vi "day 17 task 1.vi"() -> ()   [LabVIEW 2019]
uses:
  day 17/day 17 data--cluster.ctl
panel:
  out "height":i32
  out "already fallen rocks max y":i32
  out "jet pattern index":i32
  out "action":enum16{"spawn rock", "jet", "try fall"}(ring)
  out "direction of jet":string
  out "visualisation":bool[][](array[boolean])
  out "transposed array":bool[][](array[boolean])
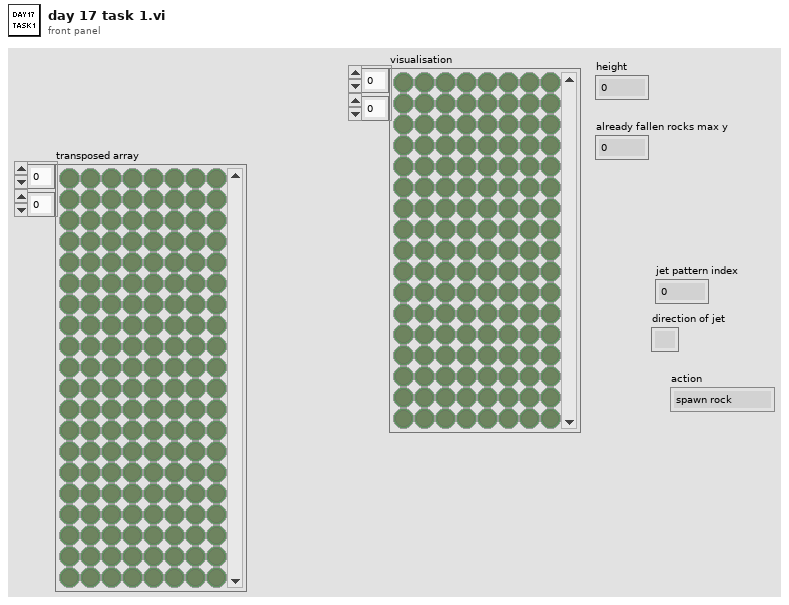
[diagram p1: front panel]
types:
  T1 = typedef "day 17 data--cluster.ctl" = cluster{"rock shape coords":cluster{cluster{"x":i32, "y":i32}[]}[], "index of next rock shape":i32, "currently falling rock's co-ords":cluster{"x":i32, "y":i32}[], "already fallen rocks' co-ords":cluster{"x":i32, "y":i32}[], "jet pattern":string, "index of next jet pattern index":i32, "next action":enum16{"spawn rock", "jet", "try fall"}, "already fallen rocks max y":i32, "no. rocks fallen":i64}
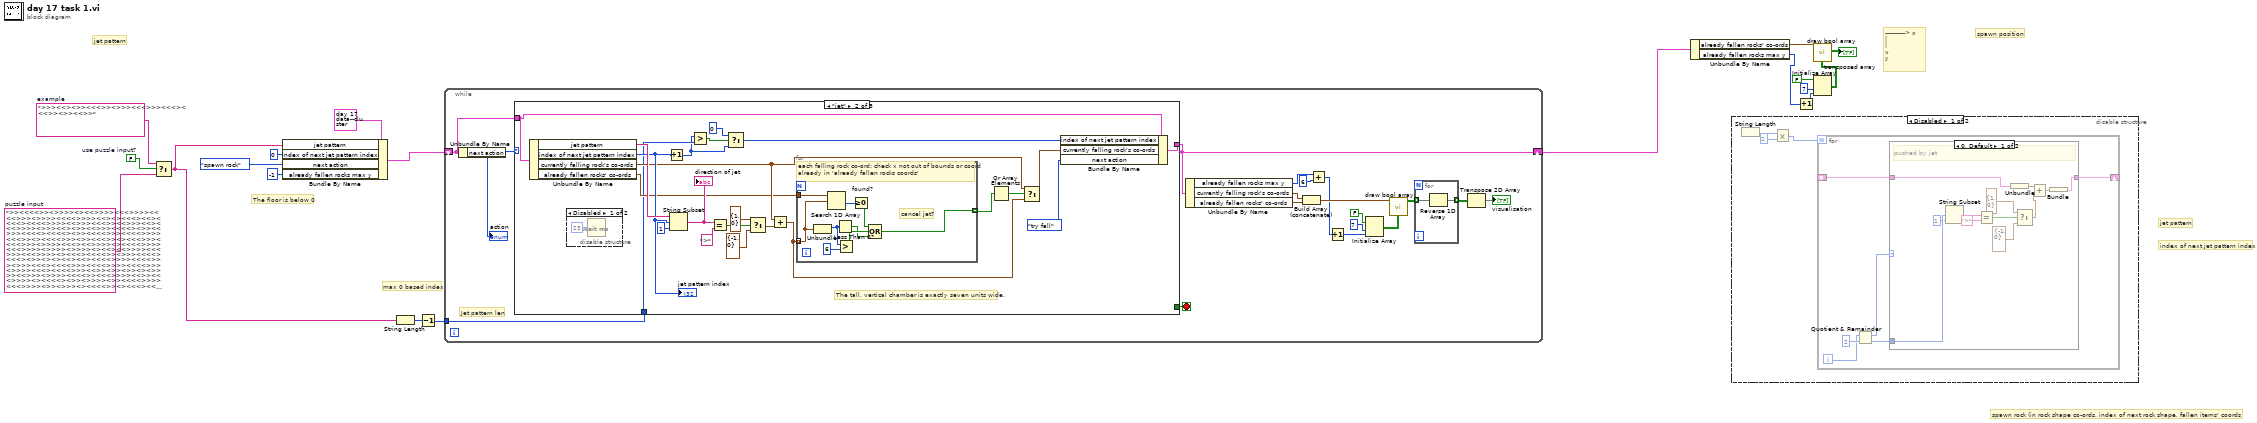
[diagram p0: block diagram]
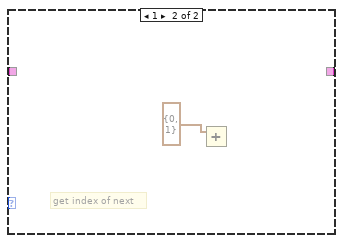
[diagram p2: hidden frame]
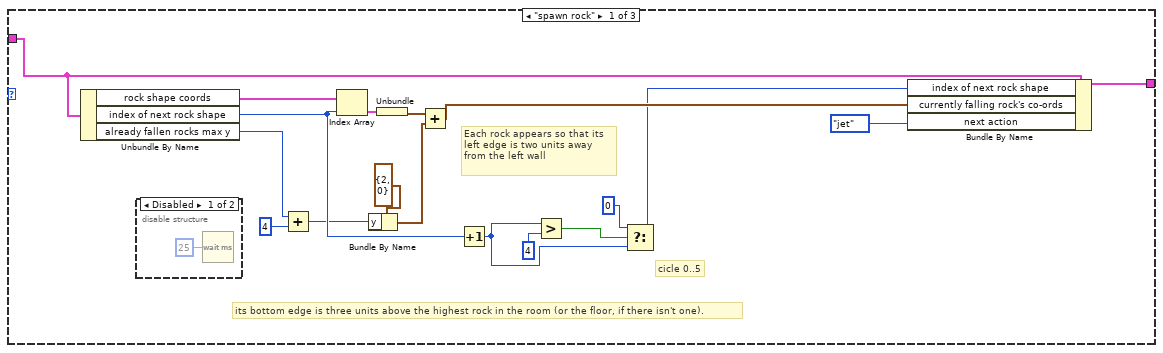
[diagram p4: hidden frame]
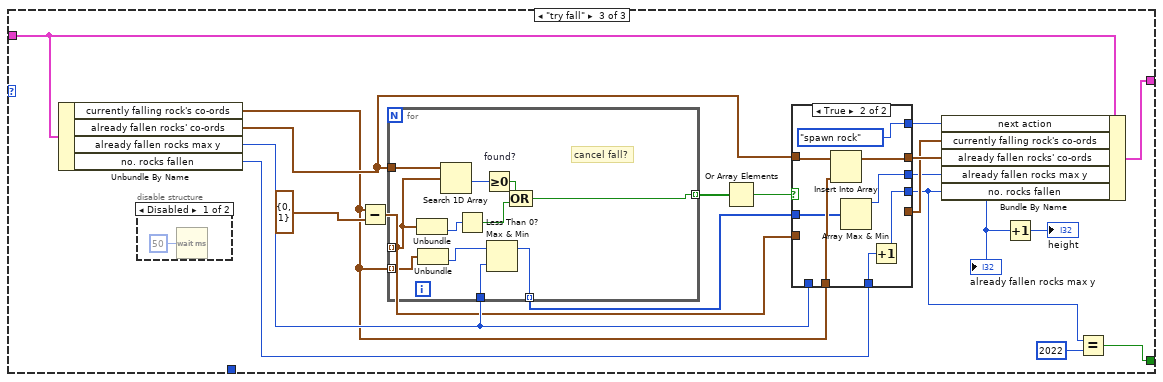
[diagram p7: hidden frame]
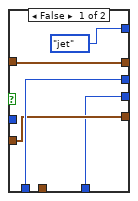
[diagram p8: hidden frame]
diagram:
  w17 = FALSE  # use puzzle input?
  w18 = ">><<<<>><>>>><><<>>>><<<>>>><<<<>>><>>>><<<<>>>><<><><<<><<><<<<><<<<>>>><<>>><<<>><<>>><<><<<>>>><>>><<><>><<>>><<<<><>><<>>><<<<><<<<><>><<<<>>><<<<>>>><<<>><><<<<>>><>><<<>><><<<>>><<<<>>><>>>><<<><<>>>><><<<<>>>><<<>>>><>>>><>>>><><<><<>>>><<<>>><<<>>>><><<<><<<<>><>>><<<<><<<><>><><><<><<><<<<>>>><<<<>>><>>><<<><<<<>>><<<<>>>><<<<>>><>>>><<<><<<<>>><<>><>><>><><>>>><<>>><>>>><<<<>><<<>>>><<>><<<>>>><><<<<><>><>>>><>><<<<>>>><<<>>>><>><>>><><<<<>><><<<><<<<>>><<><<<>>><<<<><<>>><<>><<<<><<>>>><<><>>><<><<<>>><<<<><<<<>><>>><<<>>><<<<>>>><<><<>><<<>><<>>>><<<>>>><<>><<>><<><<<<>><<<<>>><<><<<<>>><>><<>><<<<><<<><<<>>>><<<<>><>>>><<<<>><<>>><<>>>><<<<><<<><<>>><>>><<<>>>><>><<><><<<<>>>><<<<>>>><<<<><<<>>><<>><>>>><>>>><<<<>><<<<><<><>><<<<>><<<>>>><<>>>><<<<><<<>>><<<<>>><<>>><<<>>><<><<><<<>>><><<>>><<<>>>><>>>><<<><<<<><<>><><<>>>><><<<<>>><<><<<<><<<<><<<<>>>><<>><<<><<<>><<>>><<>><<<<><<><<<>>><<>><<<><>><<><<<<><<<<>><<>><<><>>><>>><<<>><<<>>>><>>><>><<><<>><><<<<><<<<>>><<<<>>><<<<><<<>>><<<>>>><<<>><<>><><<><<<<><>>>><>>>><<<<><>>><<<>><<<>>>><<<<>><<<<>><<<<>>>><>><<>>>><<<>>><<><<<>>>><<<><<><<<>>>><<<>>>><<>><<<<>>>><><<<>>><>>>><<<>>>><<>><<<<>>>><><<<>><<<>>><<>>><>>>><<>>><><<<<><>>>><><<<<>>>><<<<>><<<>>>><<<>><<<>><<<>>>><><<<<>>><<>>>><<>><><<<>>><<<>><<<>>>><>>>><<>>><<<<>>><<<>><><<<>>><<<<>>>><<>><<>>>><<<<>>><<<><>>><<<>>>><<<<>><<<<><<<<><<<<>>><<<>>><<<>>>><><>>>><>>><<>>><><>>><<>>><>><><<<>>>><<<>><<<<>>><<>>>><<>>><<<>><<<<>><>>><<<>>>><<<>>><<<>>><><><<<>>><<<>><<<>><<<<>><>>><<><>>><<>>><<>>><<<><>>><<<<>>><<<>>><<<>>><>>><<>><<>>>><><<<<>><>>>><<<<><<><<<<>>><>><>>>><<>>>><<>>>><<<>><>>><><<<<>>><><<>><<<>><<<<><<<><<<<><<<>><<>>>><<<<>>><>>><<<<><<<>><<<>>><<>>>><<<<>>>><<>>><><><<<<>>>><>>>><<<<>>><><<<><<<>>><>>><<<<><<<<><>>>><>>>><<><<<>>>><<>>><>>><<<<>>><<<<><<>>>><<<>>><<<<>>><>><<<><>>>><<>>><<<>><<<<>>>><<<>>><<<<><<<<><<>><>>><>><<<<><>>><>>>><<>><>>><<><<<><<>><<<>><>>><<<<>>>><>>>><<<<>>><<<><<<<>>>><<<<>>><<<<>>>><>>><<<>><<>>>><<<<>>>><<<<><<>>>><<<>><>>><<>><><<<<>><<<<>>><<<><<>>><>><<<><>><<>>><>>>><<>>><>>><>><<<><<>>>><<<<><<>><<<<><<<><<<<>>><<<<>>><<<>><<<<>>><<<<>>>><<><<>>><<<<><<>><<<<><<><<<<>>>><<<><<<<>><<<<><>>>><<><<<<>><>>>><><<<>>>><<<>><<<<>>>><<><<<<>><<>><<<<><<<><<>>><<>><>><<><<><>><<<<>>><<>>><>>><<<><<<<><<>>>><<>>><<>><>>>><><<<<><<>><>>><><<>>><<>>>><<<<>>><<<<>>>><<<>><<<<><<<>>><<<>><<<<><<<><><<>>>><<<>>>><<<>>>><<<>>><<>>>><<>>>><<<<>>><<>>><<<>><<>><<>>>><<<>>>><<<<><<>><>>><<<<>>>><<<><<>><>>>><>>>><>>>><<>><<<><<><>><<<>><<<<>><><<>><<>><<>>><><<<>><>><<><<<<><>>><>><<<>>>><<<>>><>>>><<>><><<>><<>>>><<<<><>>>><<>><<>>><<<>>>><<<<>><<>>><<<<>>>><>>><<<>><<<<>>>><<<<>>><<<>><<>>>><<<><<<<>><<<<>><<><<<>>><<>><<<><<<>>>><<<<>>>><<<<>><<<<>><><<>><<<<>>>><<<<>><<>>>><<>><>>>><<<><>><<><>><<>><><<><>>><<<>>>><>>><<>><>><>>>><<<<><<>><<<<><>>>><<>>><<>>><<><>>>><>><<<><<<><>>>><><<><<<<><<><<<<>>>><><<<<>>>><<<>><<>><<<<>>>><<<<>>>><<<>>>><>>><<<>>>><<<>><<<<>>>><<<>><<>>><<<<>>><<><<<<>>>><>><<<>><<>>>><<<<>>>><<>>><<<<>><><<<<>>><<<>>>><<>>>><><>>>><<>>><>>><<<>>><<<>><<<>><<<<><><<><<<<>><>>><>>><><>>><<<>>><<>><<><<<>>>><<<>>><>><><<>>>><<<><>><<<<>><<<><>>><<><<<<>>>><<>>>><<<<>><<<<>><<<<>>>><<<<>>><<<<><<<>><<>><<<<>><<><<<<>><<<<>>><<<<><<<<>>>><<><<<><<<<>>>><<>>><<<<>>>><<<<><<>>><>>><<<><<<<>><<<>>><>>>><><>>>><><>>><<<>>>><<<><>>>><<<>><<<><<>><<><><<<<><<>>><<>><<><<<>>>><<<>>><>>><>><<<<>>><<><<<<>><>>><<<>>>><<>><>>><<<>>><<<>><<<<>>>><>>><>>>><>>><<<>>><<<>>>><<<>><<<>><<<><><>>>><<<<>>>><<<<><>>><><<<<>>><<<<>>><<><><><<>><<><<<<>>><>>>><<>>><<>>>><<<>>><<<>><<<<><>>><>><<<<><<>><<<<><<<<>>>><<<>>><>>>><<<<>>>><<<<><<<<>>>><<<<>>>><<<>><<<<>>>><<>><<<>>>><<<>>>><<<<>><<<><>>>><<><>>>><<<<><>>><><<<><>>>><<>><<<<>><>><<<<>>>><<<<>><<>>><><<<><<<<>>>><>>>><<>><<<><<>>><<>><>><<>><<><<<<>><>><<<<>>>><<<<>><<<<>>><<><<>><>>><<<<>>>><<>>>><<><<>>>><<>><<>>>><<<>><<<<>>>><>>>><<<<><<<><><<<><<<<>><<<><<>><<<<>><<<<>>><<<><<<>><<>><<<>>><<><<>><<>>><<<>>>><>>><<<>>>><<>>><<<<>>>><><>>><<<<>>>><>>>><<<>>><<>>>><<<>><>><>><<<>>><<<>>>><<<>>><<<>>>><<>>>><<<><>><<>>><<<<>>>><><<<<><<>><>><>>><>>>><<>>><<<<>>><<<<><<<>>>><<<<>>>><<<<>>><>><>><<<<>>><<<<>>>><<>>>><<<<><>><<>>>><>>><<>><<<>>><<<>><<<><<<<>>>><<<<>><<>><<>>>><<<<>>>><>><<>>><<<<><<<><><<<>>><<>>><<<>>><<<>><<>>><>><<<>>>><<>>>><<<<>>>><<>><>>>><<<<><>>><<<<>>>><<>>>><<<<>>><<<<>>><<<<>><<>>><<>>>><<>>><<<><<<>>><<>>>><<<<><<>><<<<>>>><>>>><>><><<><<><<<<>><<<><<>>><>>><>>><<<<><<<<><<<<>>>><<>><>>><>>><<<><>>>><>>><>>><<<>><<<><<<>><<<<>>>><<<>>>><<<>><>><<>><<<>>>><<<<>>>><<<>>><><>><<><<<>><<<<>>><<>><<>><<<<>>><<<>>>><<>>>><<<<>>><<<>>><<<><>>>><<<<>><>><<<<>>>><<>>><<<>><><<<><<<<><>>>><>><><>><<<>>>><<<>>><<>>>><><<<<><<<>><<<<>>><<<><<><<<>><>>><><<<>>>><<<<>>>><<<>><>><<<>><<<>><<><<<<>>>><<>>><<<>>><>>>><<<>><<<<>>><<><>><<<<><<<<>><<<>><><>><<<><<<><><<<<>>>><<<><<<<><<<>>>><<>><<><><>>>><><>>><<>>><<<>><<<><<<<>>>><<<><<>><<<<>>><>><<><<>>>><<<>>><<<><<<>>><><<<<>>>><<><>><>>><<>>><<>>>><<>>><<>>>><>><><<<<>><>>><<<>>><<<>><<>>><<<<>><>>><<>>>><<<>>><>>><<<>><<<><<<>>><<><<<>>>><<>><<<<>>><<<>>><<<>>>><>><<<>>><<<<>>>><<><>>>><>>>><<<<>><<<>>>><>>>><<<>><<<<>><<><<>>>><<<<>>><<<<>>><<>><<<<>><<>>><<>>>><>><<>>><<>>>><>>>><>>><<<><<>><<<<>>>><<<>><<<<>>>><<<>><<<><<<>>><<<>><>>><<<<>>>><>>>><<<>><<<<>>><>>>><>><<><><><<<<>>>><<<<><>>><<>><<<>><<<>><<><<>><>><<<><<<>><<<>>><<<>><<>>><<<>>><<<<><>>><>>>><><<>>>><>>>><<<<>>><>>><<<<>>><>>>><>>>><<<<>>>><<>>>><<<>>><<>><<>>><<>>>><<>><>>>><<<>><<<><<><<<>><<<<>>><<>>>><<<<><>><<<>>>><<<>>>><<>><<>>>><<><>><>>><<<<>><<<>>>><<<>>>><<<<>>>><>>>><>>><<<<>>>><<<<><<>>>><<<<>>><<<<>><<>><>>><<<>><<<><<<<>>><><>><>>>><><<><<<<>>>><><<<>><<>>><<<<>>><<<<><>>><<>><>><<<><><>><<>>><<><><<><>><<>>>><<<<><<>><<<><<<><<>>><<<<><>><>>><<<><<<>><<><<<>><<<<>>>><<<>>><<>>>><><>><>>>><>>><>>>><>>><<<<>>>><<<>>><<<<>>>><>><<<<><<>><>><<>>><<<<>>>><<<>>><<<>><<<>><<>><<<<><>>>><>>>><<>>><<<><>><>><<<<>>><>>>><>><<>>>><<<<>><>>><<>>><<<<>>>><<><<<<>>>><<><<>><><>>>><>>><>>>><>>><<><>>><<>>><<<>>><<<<>>>><>>><<>><>><>>>><<>><<<>>><<<>>>><>><<>>><<>>><<><<>>>><<<<>>>><>><<<<>>>><<<<>>>><<>><<>>>><<<<>>>><<<<>><>>><>>>><<<>><>>>><<<><<>>>><<>>><<>>>><<><<<><<<<><<<>>><<>>><<<>>>><<><<<><><<>><<<<><<<<>>><<><<<<>><<<<>>>><<<>>>><<<>><<<<>>><>>><<<<>>><<<>>><<<<>><<<<>>><<>>><<<>><<<<>>><>>><<<>><<<<><<<<>>><<><<<<>>>><<<>>>><<>>><<><<<>>>><>>>><<>>>><>><<>><<>>>><<<<>>><<<>>>><<><<<><>><<<<>>><><>><<>>><<<>><<<>>><<<<><<<>>><<<<>>><<<<>><<><<<<>>>><<<><>><<>><>>>><>><<>><><<<>><<<>><<<<>>>><<<>>><<><<>>>><<>>>><<>>><<>><<<<>>>><<<<>><<>>>><<<>>>><<<<>>><<><<<<>>>><<<><>>><<<>><><>>>><><<<>>>><<<<>><<>><<<>><<><<><<<<>><><<<<>>><<><<>><<<>>>><<<>>><<>>><<<<>><<><<<<>>><<<<><><<<>>><<<><<<<>>><<<<>>><<<<>>><<<<>>><<>>><<<<>>><>><<<>><<<<>>>><><>>>><<><<><<<<>><><<<>>><><<<><<<>>>><<>><<<<>>><<<<><<<>>>><<>>>><<<<>><<<>>>><>>><<<>>>><<<>>>><<<>>><>>>><<<<>><>><<>><><<<<><<<>>>><<<>>><>>>><>>>><<<><<<>>><<>>>><>>><><<<<>><<>>><<<>><<>>><<<<><<<<>>>><<><<<><>>>><<<>>><<>>>><<<<>>>><<<<>>>><>><<<<>>><>>>><<>>>><<<><<>><<<>>><<<><<>>><<<<>>><<<<><<>>>><<>><<<>>><<<<>><<><<<<>>>><<><<>>><<<>>>><<<><<>><<<>>>><<><<>>>><>><<<<>>>><<>><>><<>>><<<><<<<><<<<>>><>><><>>><<<>>><<>><><<>><<<>>><<<>><<<<>>><<<<><<<><>><>>><<<<>>>><<<<>><<<<>><>>>><>>>><>>>><<<<>><>>>><<>><<<>>><<>><><>>>><<><<<<>><<>>><<>>><<>>><<<<>>>><<<<>><<<>>><<><<<<>><<<<>><<><>>>><<<>>>><<<><<>><<<<>>><<<<><>>>><<<<>>>><<>>>><<>><>>><>>><<><<<<>><<<<>><><<>><>><>>><<><<<>>>><<<>>><<<<>>>><<><<><>>><<<<><><<>>>><<<<>><<<<>><<>><<>>>><<>>>><<>>><<<>>>><<>>>><<<<>><>><>><<>>>><<<>>>><<<<>><<<>>><<>>><<<<>>>><>>>><<>>><<>>>><<<<><<>>><<<<>><<<>>>><><<<>>>><<<>>><<<<>>><<<<><<><<><<<<>>><<<>><>>><>><<<<>>><<<<>>><<><<<<>>><>>><<<>>><<>>>><<<>><<>>>><<><<<>><<<>>><<<<>>>><<<<>>>><>>><<>>><<<><<<>>>><<>>>><<><<<><>>><<>><<><<<<>>><>><>>><<<><><<><<<>>><<<><><<>>><<><<>><>>>><>><<<>>><<<>>>><<<>><<<<>>><>>>><<<<>><<<<><<<<><<<><>><<<<><<>>><<<<>>>><<<>>><<<>>>><>>>><<<<><<<<><<<<><<>><><<<<>>>><<<<>><<<>>>><<<>><<<>>>><<<>>>><<<><<>>><>><<<>>><<>><<<>>><>><<<>>><<<<>><>>>><>>>><><>>>><<<>>>><<<<><<><<><>><>>>><><<>><<<>>><<<<><>><<>><>>>><><<<>>>><<<>>>><<>>>><>>><>>>><<<>>><>><<<<><<<<>>>><<<<>><<<>>><<>>><<<<>>><<<>><>>><<><<<><<>>><<>><<>>><<<<>>><<<>>>><<<<><<<<>>>><<<>>>><<<<>>>><<><>><<<><><<>>>><><<<>>><<>>><<>>>><<<<>>><<<>>><<<<>>>><<>>><<<>><>>>><<>><<<><<><<<>><<<<>>><><>>>><><<><><<>>>><<>>>><>><><>>>><<<><<<<>>>><<<>><<<>><<<>>><<<>><<<>>><<<><<<>>>><<<<><<>><<<>>><<<<>>>><<<<>><<<<>>>><>>><<><<>>><><<<>><<><<<<>>><<<<>>><<<<>><<<>>><<<<><>><<>>><<<<>>><<<>><<<>><<<>>><><<<>><<>>><>><>><<>>><<<>>>><<<>>>><<>>><>><>><<>>><<>>>><<>>><><<<>><<>>><<>><<>><<<<>>>><>>>><<>><<<><<>><<<<>>>><<<<>><<>><>><<<>><<<<><<><<>>>><<>>>><<<>><<<<>>><<<<><<<>><<<>><>>>><>>>><<><>>>><<<>>><<<<>>><<<>><<<<>>><<<><<<>>><>>><<<<>><<>>>><<>><<<>><<<>>>><<<<>><<>>><<<<>><<>>>><<><<<>>><<<<>><>>>><<<<>>>><>>>><>>><<<>>><<<>>><>><>>>><<<<>>><<<<>>><<>>><>>><><<<>><<<<>>>><>>>><<<>><>>>><<>>>><<<><<>>><<<<>>>><<><>>><<<<>><<<>>><>>><<>>><<<><>>><<><<<>>>><<<<>><>>>><<><<>><>>><<>><>>>><<<<>>>><<<<>>><<>><<><><<<<>>>><<>>><<<>>>><<<>>><<<<>><<<<>><<>>>><<<<><<>>><<<><<<>><<<<>>><<<<>><<<>>><<><<>><<<<>>><<<<>>><<><>>><<<><<<<>>>><<<<>>>><>><>>><<<>>>><<<><<>>><<>><<<<>>><<<<><<<><<<>>><<>><>><>>>><>>>><><<<><><<<<><>>>><<>>><>>>><<>>><<<<>>>><<>>><>>>><<<>><><<>>>><<>>><<<>>><<<><<<>><<<>>><<<>>><<><<>><<<>>><<<<>>><<>>><>>><<<<>>><<>>>><<<><<<<>>><>><<<<>><>>><<>><>>>><<><<<<>>><<<<>><<>>><<<>>>><<<<>>><<<>><>>>><<<<>>><>>>><<>><>>><><>>><>>>><<<<>><<<><><<>><>><<<><<>>><<>>><<>><<<>>><<<<>><>><<<>><<<<>>>><<>>><>><<<<>>><<<><<>><>>>><<><<>>><<<>><><<<>>>><<<<><<<<>>>><<<>>><<<><>>><<<>>><<<<>><<<><<>>>><<<<>>>><<>><><<>>><<<<>>><>><<<<>>><>>>><>>><<<<>>><<><<<>>>><<<><<<>>><<<<>>><<<>>>><<<>><>><<<<>>>><<<<>><<<><>><<<><<>>>><<<>><<<<>>><<<<>>>><>><<<>>><<>>><<><<>><<<<>><<<<>><>><<<>>>><<<>>><<<>>><<>>>><<>>>><<>><<>><<>><<>><<>><<><>><>>><<<>>><<><<<<>>>><><<<>><<<<>>>><>><>>>><<><<<><>>"  # puzzle input
  w19 = ">>><<><>><<<>><>>><<<>>><<<><<<>><>><<>>"  # example
  # "The floor is below 0"
  # "max 0 based index"
  # "spawn rock (in rock shape co-ords, index of next rock shape, fallen items' coords"
  # "index of next jet pattern index"
  # "jet pattern"
  # "spawn position"
  # "----------> x\n|\n|\nv\ny"
  # "jet pattern"
  n1 = Select(t=w19, s=w17, f=w18) -> (s? t:f=w13:string)
  n2 = Bundle By Name(cluster=T1 {"rock shape coords"=[{[{"x"=0, "y"=0}, {"x"=1, "y"=0}, {"x"=2, "y"=0}, {"x"=3, "y"=0}]}, {[{"x"=1, "y"=0}, {"x"=0, "y"=1}, {"x"=1, "y"=1}, {"x"=2, "y"=1}, {"x"=1, "y"=2}]}, {[{"x"=0, "y"=0}, {"x"=1, "y"=0}, {"x"=2, "y"=0}, {"x"=2, "y"=1}, {"x"=2, "y"=2}]}, {[{"x"=0, "y"=0}, {"x"=0, "y"=1}, {"x"=0, "y"=2}, {"x"=0, "y"=3}]}, {[{"x"=0, "y"=0}, {"x"=0, "y"=1}, {"x"=1, "y"=0}, {"x"=1, "y"=1}]}], "index of next rock shape"=0, "currently falling rock's co-ords"=[], "already fallen rocks' co-ords"=[], "jet pattern"="", "index of next jet pattern index"=0, "next action"=enum."spawn rock", "already fallen rocks max y"=0, "no. rocks fallen"=0}, "jet pattern"=w13, "index of next jet pattern index"=0, "next action"=enum16{"spawn rock", "jet", "try fall"}."spawn rock", "already fallen rocks max y"=-1) -> (w12:T1)
  n3 = String Length(string=w13) -> (length=w14:i32)
  n4 = Decrement(x=w14) -> (x-1=w11:i32)
  n5 = while {
    shift-right: [w31] -> w9
    shift-left: w12 -> [w36]
    tunnel: w11 -> [w21]
    stop <- w20 stop-if-true
    # "Jet pattern len"
    n6 = Unbundle By Name(w36) -> ("next action"=w37:enum16{"spawn rock", "jet", "try fall"})
    "action" <- w37
    n7 = case shown="\"jet\"" w37 {
      tunnel: w36 -> [w56 w74 w109]
      tunnel: [w54 w73 w110] -> w31
      tunnel: w21 -> [_ w63 _]
      tunnel: [_ _ w94] -> w20
      frame "spawn rock" {
        # "cicle 0..5"
        # "its bottom edge is three units above the highest rock in the room (or the floor, if there isn't one)."
        # "Each rock appears so that its left edge is two units away from the left wall"
        n8 = Unbundle By Name(w56) -> ("rock shape coords"=w57:cluster{cluster{"x":i32, "y":i32}[]}[], "index of next rock shape"=w55:i32, "already fallen rocks max y"=w47:i32)
        n9 = disable-structure shown="Disabled" {
          frame Disabled {
            n10 = Wait (ms)(milliseconds to wait=u32 25) -> ()  [unwired: 1 out]
          }
          frame Enabled {
          }
        }
        n11 = Add(x=w47, y=4) -> (x+y=w45:i32)
        n12 = Index Array(array=w57, index=w55) -> (element=w52:cluster{cluster{"x":i32, "y":i32}[]})
        n13 = Bundle By Name(cluster=cluster{"x":i32, "y":i32} {"x"=2, "y"=0}, "y"=w45) -> (w48:cluster{"x":i32, "y":i32})
        n14 = Unbundle(w52) -> (w51:cluster{"x":i32, "y":i32}[])
        n15 = Add(x=w51, y=w48) -> (x+y=w50:cluster{"x":i32, "y":i32}[])
        n16 = Increment(x=w55) -> (x+1=w42:i32)
        n17 = Greater?(x=w42, y=4) -> (0:w43:bool)
        n18 = Select(t=0, s=w43, f=w42) -> (s? t:f=w40:i32)
        n19 = Bundle By Name(cluster=w56, "index of next rock shape"=w40, "currently falling rock's co-ords"=w50, "next action"=enum16{"spawn rock", "jet", "try fall"}."jet") -> (w54:T1)
      }
      frame "jet" {
        # "The tall, vertical chamber is exactly seven units wide."
        n20 = Unbundle By Name(w74) -> ("jet pattern"=w76:string, "index of next jet pattern index"=w75:i32, "currently falling rock's co-ords"=w67:cluster{"x":i32, "y":i32}[], "already fallen rocks' co-ords"=w65:cluster{"x":i32, "y":i32}[])
        "jet pattern index" <- w75
        n21 = disable-structure shown="Disabled" {
          frame Disabled {
            n22 = Wait (ms)(milliseconds to wait=u32 25) -> ()  [unwired: 1 out]
          }
          frame Enabled {
          }
        }
        n23 = Increment(x=w75) -> (x+1=w60:i32)
        n24 = String Subset(string=w76, offset (0)=w75, length (rest)=1 ("length (rest)")) -> (substring=w80:string)
        "direction of jet" <- w80
        n25 = Greater?(x=w60, y=w63) -> (0:w62:bool)
        n26 = Equal?(x=w80, y=">") -> (x = y?=w78:bool)
        n27 = Select(t=0, s=w62, f=w60) -> (s? t:f=w59:i32)
        n28 = Select(t=cluster{"x":i32, "y":i32} {"x"=1, "y"=0}, s=w78, f=cluster{"x":i32, "y":i32} {"x"=-1, "y"=0}) -> (s? t:f=w70:cluster{"x":i32, "y":i32})
        n29 = Add(x=w67, y=w70) -> (x+y=w66:cluster{"x":i32, "y":i32}[])
        n30 = for {
          tunnel: w66 -> [w90] mode=indexing
          tunnel: [w83] -> w69 mode=indexing
          tunnel: w65 -> [w91]
          # "cancel jet?"
          # "each falling rock co-ord: check x not out of bounds or coord already in 'already fallen rocks coords'"
          n31 = Unbundle(w90) -> ("x"=w86:i32)  [unwired: 1 out]
          n32 = Search 1D Array(1D array=w91, element=w90) -> (index of element=w89:i32)  [unwired: 1 in]
          n33 = Less Than 0?(x=w86) -> (x < 0?=w84:bool)
          n34 = Greater?(x=w86, y=6) -> (0:w88:bool)
          n35 = Greater Or Equal To 0? "found?"(x=w89) -> (x >= 0?=w85:bool)
          n36 = Compound Arithmetic op=OR(w85, w88, w84) -> (w83:bool)
        }
        n37 = Or Array Elements(Boolean array=w69) -> (logical OR=w68:bool)
        n38 = Select(t=w67, s=w68, f=w66) -> (s? t:f=w64:cluster{"x":i32, "y":i32}[])
        n39 = Bundle By Name(cluster=w74, "index of next jet pattern index"=w59, "currently falling rock's co-ords"=w64, "next action"=enum16{"spawn rock", "jet", "try fall"}."try fall") -> (w73:T1)
      }
      frame "try fall" {
        n40 = Unbundle By Name(w109) -> ("currently falling rock's co-ords"=w98:cluster{"x":i32, "y":i32}[], "already fallen rocks' co-ords"=w104:cluster{"x":i32, "y":i32}[], "already fallen rocks max y"=w103:i32, "no. rocks fallen"=w97:i64)
        n41 = disable-structure shown="Disabled" {
          frame Disabled {
            n42 = Wait (ms)(milliseconds to wait=u32 50) -> ()  [unwired: 1 out]
          }
          frame Disabled {
          }
        }
        n43 = Subtract(x=w98, y=cluster{"x":i32, "y":i32} {"x"=0, "y"=1}) -> (x-y=w101:cluster{"x":i32, "y":i32}[])
        n44 = for {
          tunnel: w101 -> [w133] mode=indexing
          tunnel: [w124] -> w107 mode=indexing
          tunnel: w104 -> [w134]
          tunnel: w103 -> [w130]
          tunnel: [w129] -> w102 mode=indexing
          tunnel: w98 -> [w126] mode=indexing
          # "cancel fall?"
          n45 = Unbundle(w133) -> ("y"=w128:i32)  [unwired: 1 out]
          n46 = Unbundle(w126) -> ("y"=w125:i32)  [unwired: 1 out]
          n47 = Search 1D Array(1D array=w134, element=w133) -> (index of element=w132:i32)  [unwired: 1 in]
          n48 = Less Than 0?(x=w128) -> (x < 0?=w127:bool)
          n49 = Greater Or Equal To 0? "found?"(x=w132) -> (x >= 0?=w131:bool)
          n50 = Max & Min(x=w125, y=w130) -> (max(x,y)=w129:i32)  [unwired: 1 out]
          n51 = Compound Arithmetic op=OR(w131, w127) -> (w124:bool)
        }
        n52 = Or Array Elements(Boolean array=w107) -> (logical OR=w106:bool)
        n53 = case shown="True" w106 {
          tunnel: [enum16{"spawn rock", "jet", "try fall"}."jet" ("next action") enum16{"spawn rock", "jet", "try fall"}."spawn rock" ("next action")] -> w105
          tunnel: w98 -> [_ w121]
          tunnel: [w112 _] -> w99
          tunnel: w104 -> [w114 w122]
          tunnel: [w114 w120] -> w100
          tunnel: w103 -> [w113 _]
          tunnel: [w113 w118] -> w93
          tunnel: w102 -> [_ w119]
          tunnel: w101 -> [w112 _]
          tunnel: [w111 w116] -> w96
          tunnel: w97 -> [w111 w117]
          frame False {
          }
          frame True {
            n54 = Insert Into Array(array=w122, new element=w121) -> (w120:cluster{"x":i32, "y":i32}[])  [unwired: 1 in]
            n55 = Array Max & Min(array=w119) -> (max value=w118:i32)  [unwired: 3 out]
            n56 = Increment(x=w117) -> (x+1=w116:i64)
          }
        }
        "already fallen rocks max y" <- w93
        n57 = Bundle By Name(cluster=w109, "next action"=w105, "currently falling rock's co-ords"=w99, "already fallen rocks' co-ords"=w100, "already fallen rocks max y"=w93, "no. rocks fallen"=w96) -> (w110:T1)
        n58 = Increment(x=w93) -> (x+1=→"height":i32)
        n59 = Equal?(x=w96, y=2022) -> (x = y?=w94:bool)
      }
    }
    n60 = Unbundle By Name(w31) -> ("already fallen rocks max y"=w27:i32, "currently falling rock's co-ords"=w30:cluster{"x":i32, "y":i32}[], "already fallen rocks' co-ords"=w29:cluster{"x":i32, "y":i32}[])
    n61 = Build Array (concatenate)(w30, w29) -> (w28:cluster{"x":i32, "y":i32}[])
    n62 = Add(x=w27, y=6) -> (x+y=w25:i32)
    n63 = Increment(x=w25) -> (x+1=w34:i32)
    n64 = Initialize Array(FALSE, 7 ("dimension size"), w34) -> (w35:bool[][])
    n65 = call "draw bool array.vi"("Array in"=w35, "array with duplicates removed"=w28) -> ("Array out"=w24:bool[][])  [unwired: 8 in, 1 out]
    n66 = for {
      tunnel: w24 -> [w39] mode=indexing
      tunnel: [w38] -> w23 mode=indexing
      n67 = Reverse 1D Array(array=w39) -> (reversed array=w38:bool[])
    }
    n68 = Transpose 2D Array(2D array=w23) -> (transposed array=→"visualisation":bool[][])
  }
  n69 = Unbundle By Name(w9) -> ("already fallen rocks' co-ords"=w8:cluster{"x":i32, "y":i32}[], "already fallen rocks max y"=w4:i32)
  n70 = disable-structure shown="Disabled" {
    frame Disabled {
      n71 = String Length() -> (length=w138:i32)  [unwired: 1 in]
      n72 = Multiply(x=w138, y=2) -> (x*y=w136:i32)
      n73 = for {
        N: w136 -> [_]
        shift-right: [w139] -> _
        shift-left: _ -> [w140]
        i -> [w141]
        n74 = Quotient & Remainder(x=w141, y=2) -> (x-y*floor(x/y)=w144:i32, floor(x/y)=w143:i32)
        n75 = case shown="0, Default" w144 {
          tunnel: w143 -> [w156 _]
          tunnel: w140 -> [w149 _]
          tunnel: [w145 _] -> w139
          frame 0, Default {
            # "pushed by jet"
            n76 = String Subset(offset (0)=w156, length (rest)=1 ("length (rest)")) -> (substring=w154:string)  [unwired: 1 in]
            n77 = Equal?(x=w154, y=">") -> (x = y?=w152:bool)
            n78 = Unbundle(w149) -> (w148:cluster{"x":i32, "y":u32})
            n79 = Select(t=cluster{"x":i32, "y":u32} {"x"=1, "y"=0}, s=w152, f=cluster{"x":i32, "y":u32} {"x"=-1, "y"=0}) -> (s? t:f=w147:cluster{"x":i32, "y":u32})
            n80 = Add(x=w148, y=w147) -> (x+y=w146:cluster{"x":i32, "y":u32})
            n81 = Bundle(w146) -> (w145:cluster{cluster{"x":i32, "y":u32}})  [unwired: 1 in]
          }
          frame 1 {
            # "get index of next"
            n82 = Add(x=cluster{"x":i32, "y":i32} {"x"=0, "y"=1}) -> ()  [unwired: 1 in, 1 out]
          }
        }
      }
    }
    frame Enabled {
    }
  }
  n83 = Increment(x=w4) -> (x+1=w5:i32)
  n84 = Initialize Array(FALSE, 7 ("dimension size"), w5) -> (w3:bool[][])
  n85 = call "draw bool array.vi"("Array in"=w3, "array with duplicates removed"=w8) -> ("transposed array"=→"transposed array":bool[][])  [unwired: 8 in, 1 out]
